vi "Template - Labview.vi"() -> ()   [LabVIEW 2017]
panel:
  out "Tempo\nTOTAL":string
  out "Tempo\nValidação":string
  out "Tempo\n Torno":string
  out "Tempo \nArmazem":string
  out "Y_Ctrg":bool
  out "Z_Ctrg":bool
  out "X_Ctrg":bool
  out "Y 1":bool
  out "Y 0":bool
  out "Z3":bool
  out "Z2":bool
  out "Z1":bool
  out "Z0":bool
  out "X 3":bool
  out "X 2":bool
  out "X 1":bool
  out "X 0":bool
  out "Medição Peça":string
  out "OK":bool
  out "Nok":bool
  out "Status":bool
  out "Robô":bool
  out "Torno":bool
  out "Visão":bool
  out "Armazem":bool
  out "Valvula 4":bool
  out "Sensor 4":bool
  out "Valvula 1":bool
  out "Sensor 1":bool
  out "Esteira 4":bool
  out "Esteira 2":bool
  out "Esteira 3":bool
  out "Esteira 1":bool
  in  "START":bool caption="OK Button"
  in  "Blank Button 74":bool
  in  "Blank Button 73":bool
  in  "Blank Button 72":bool
  in  "Blank Button 71":bool
  in  "Blank Button 70":bool
  in  "Blank Button 69":bool
  in  "Blank Button 68":bool
  in  "Blank Button 67":bool
  in  "Blank Button 66":bool
  in  "Blank Button 65":bool
  in  "Blank Button 64":bool
  in  "Blank Button 63":bool
  in  "Blank Button 62":bool
  in  "Blank Button 61":bool
  in  "Blank Button 60":bool
  in  "Blank Button 59":bool
  in  "Blank Button 58":bool
  in  "Blank Button 57":bool
  in  "Blank Button 56":bool
  in  "Blank Button 55":bool
  in  "Blank Button 54":bool
  in  "Blank Button 53":bool
  in  "Blank Button 52":bool
  in  "Blank Button 51":bool
  in  "Blank Button 50":bool
  # "Imagem"
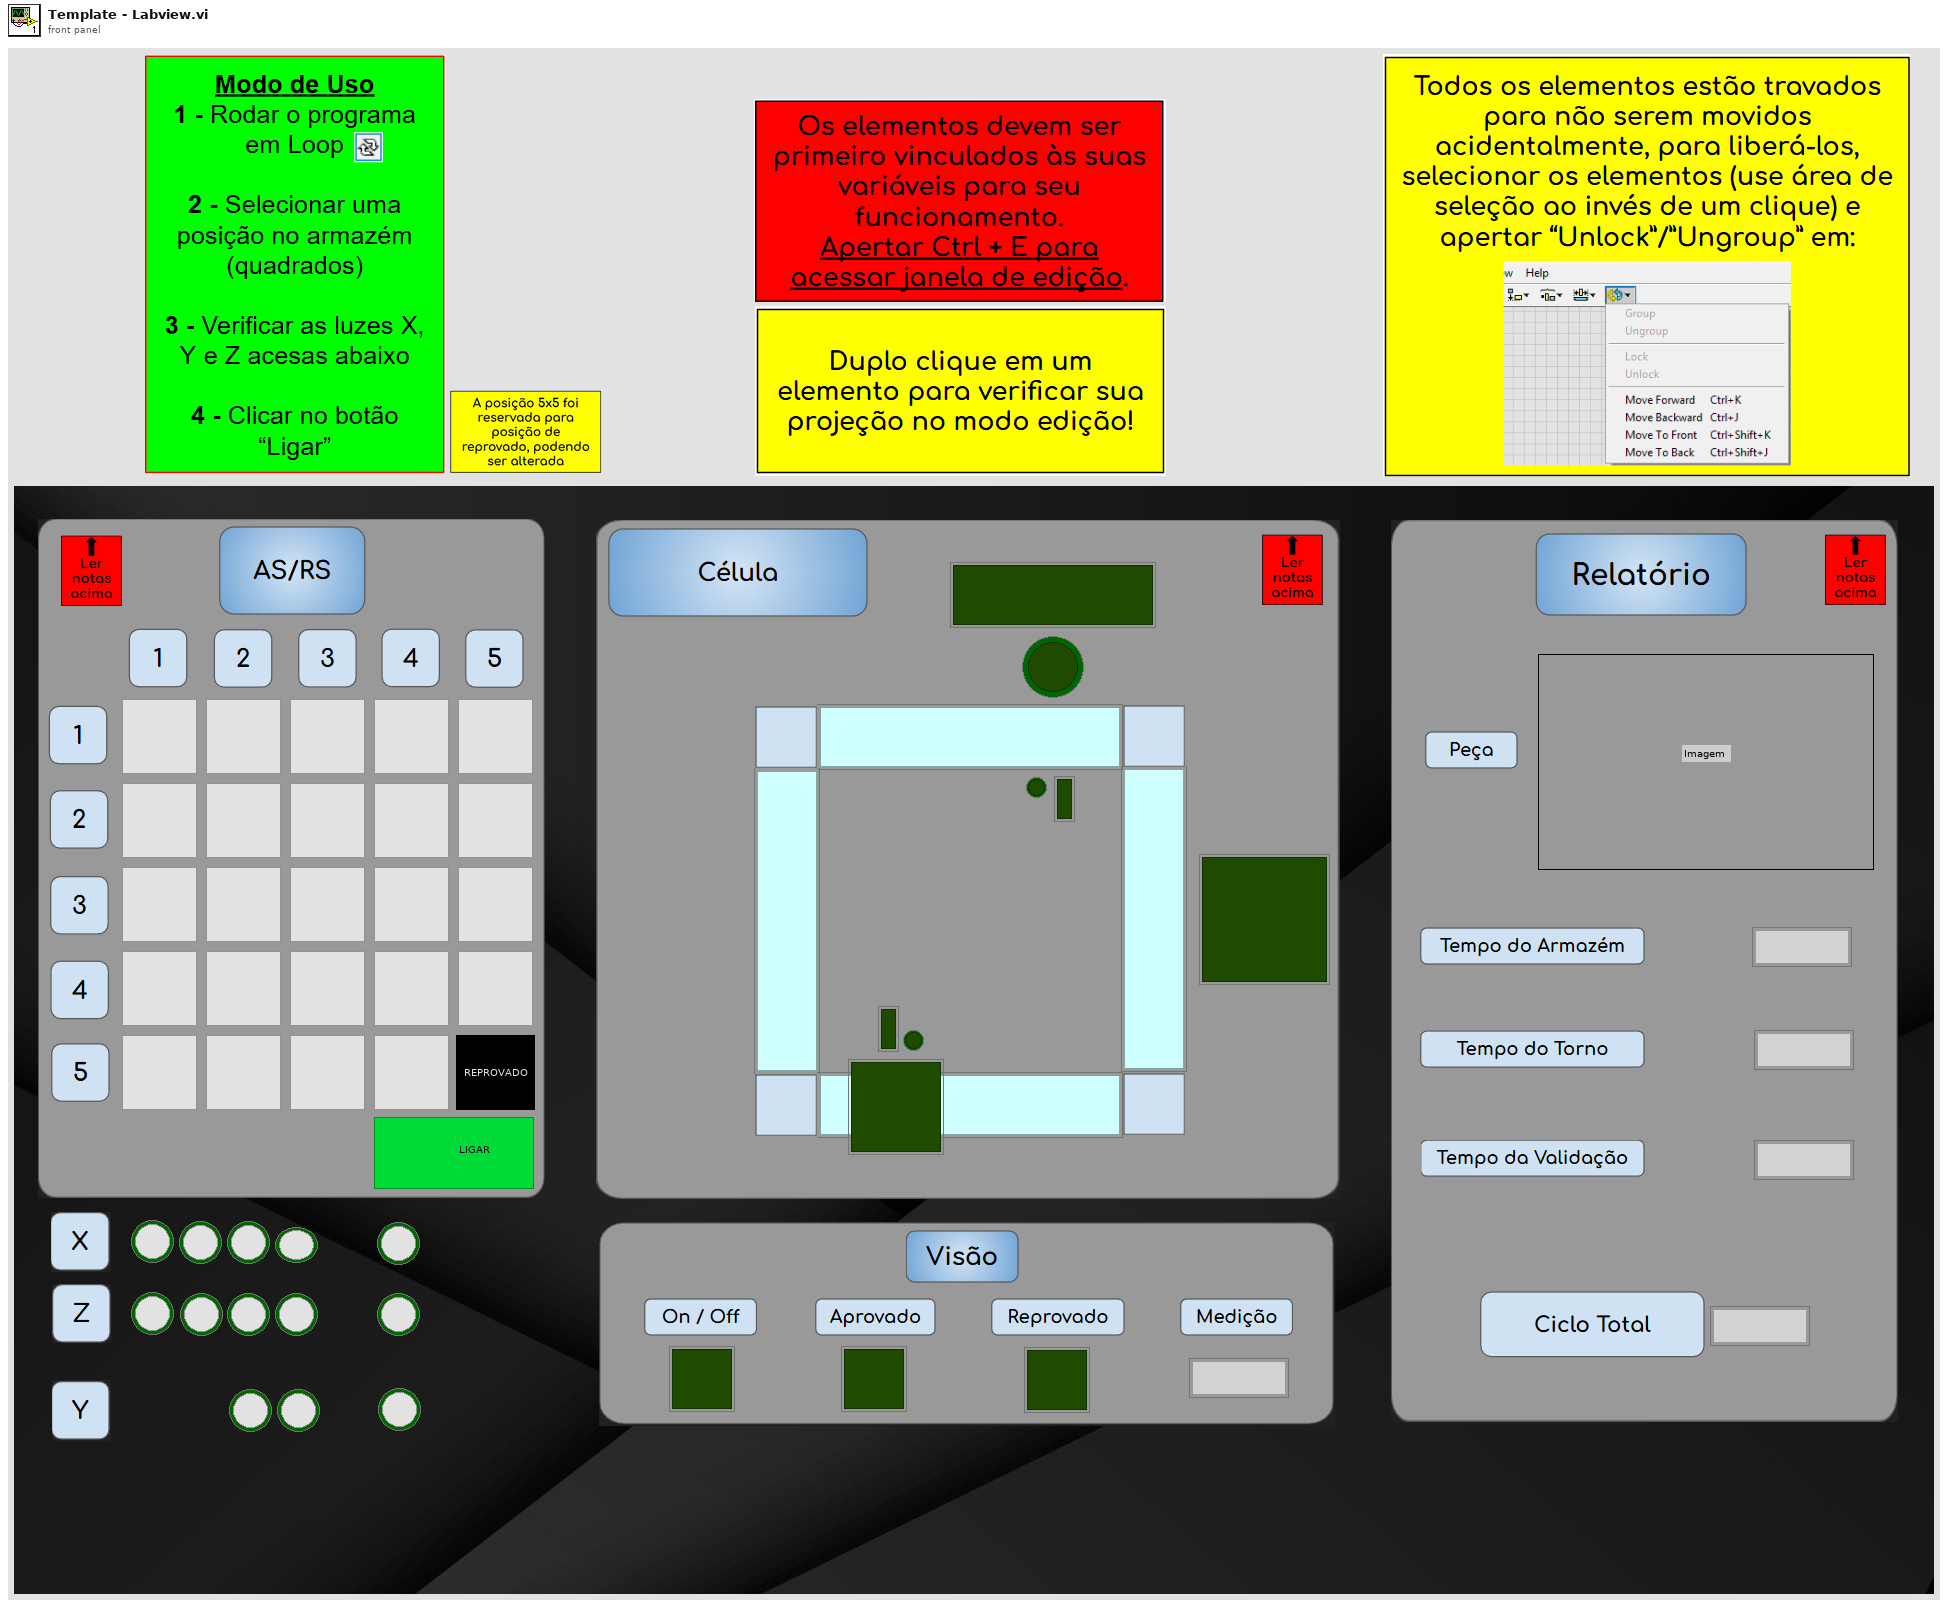
[diagram p1: front panel]
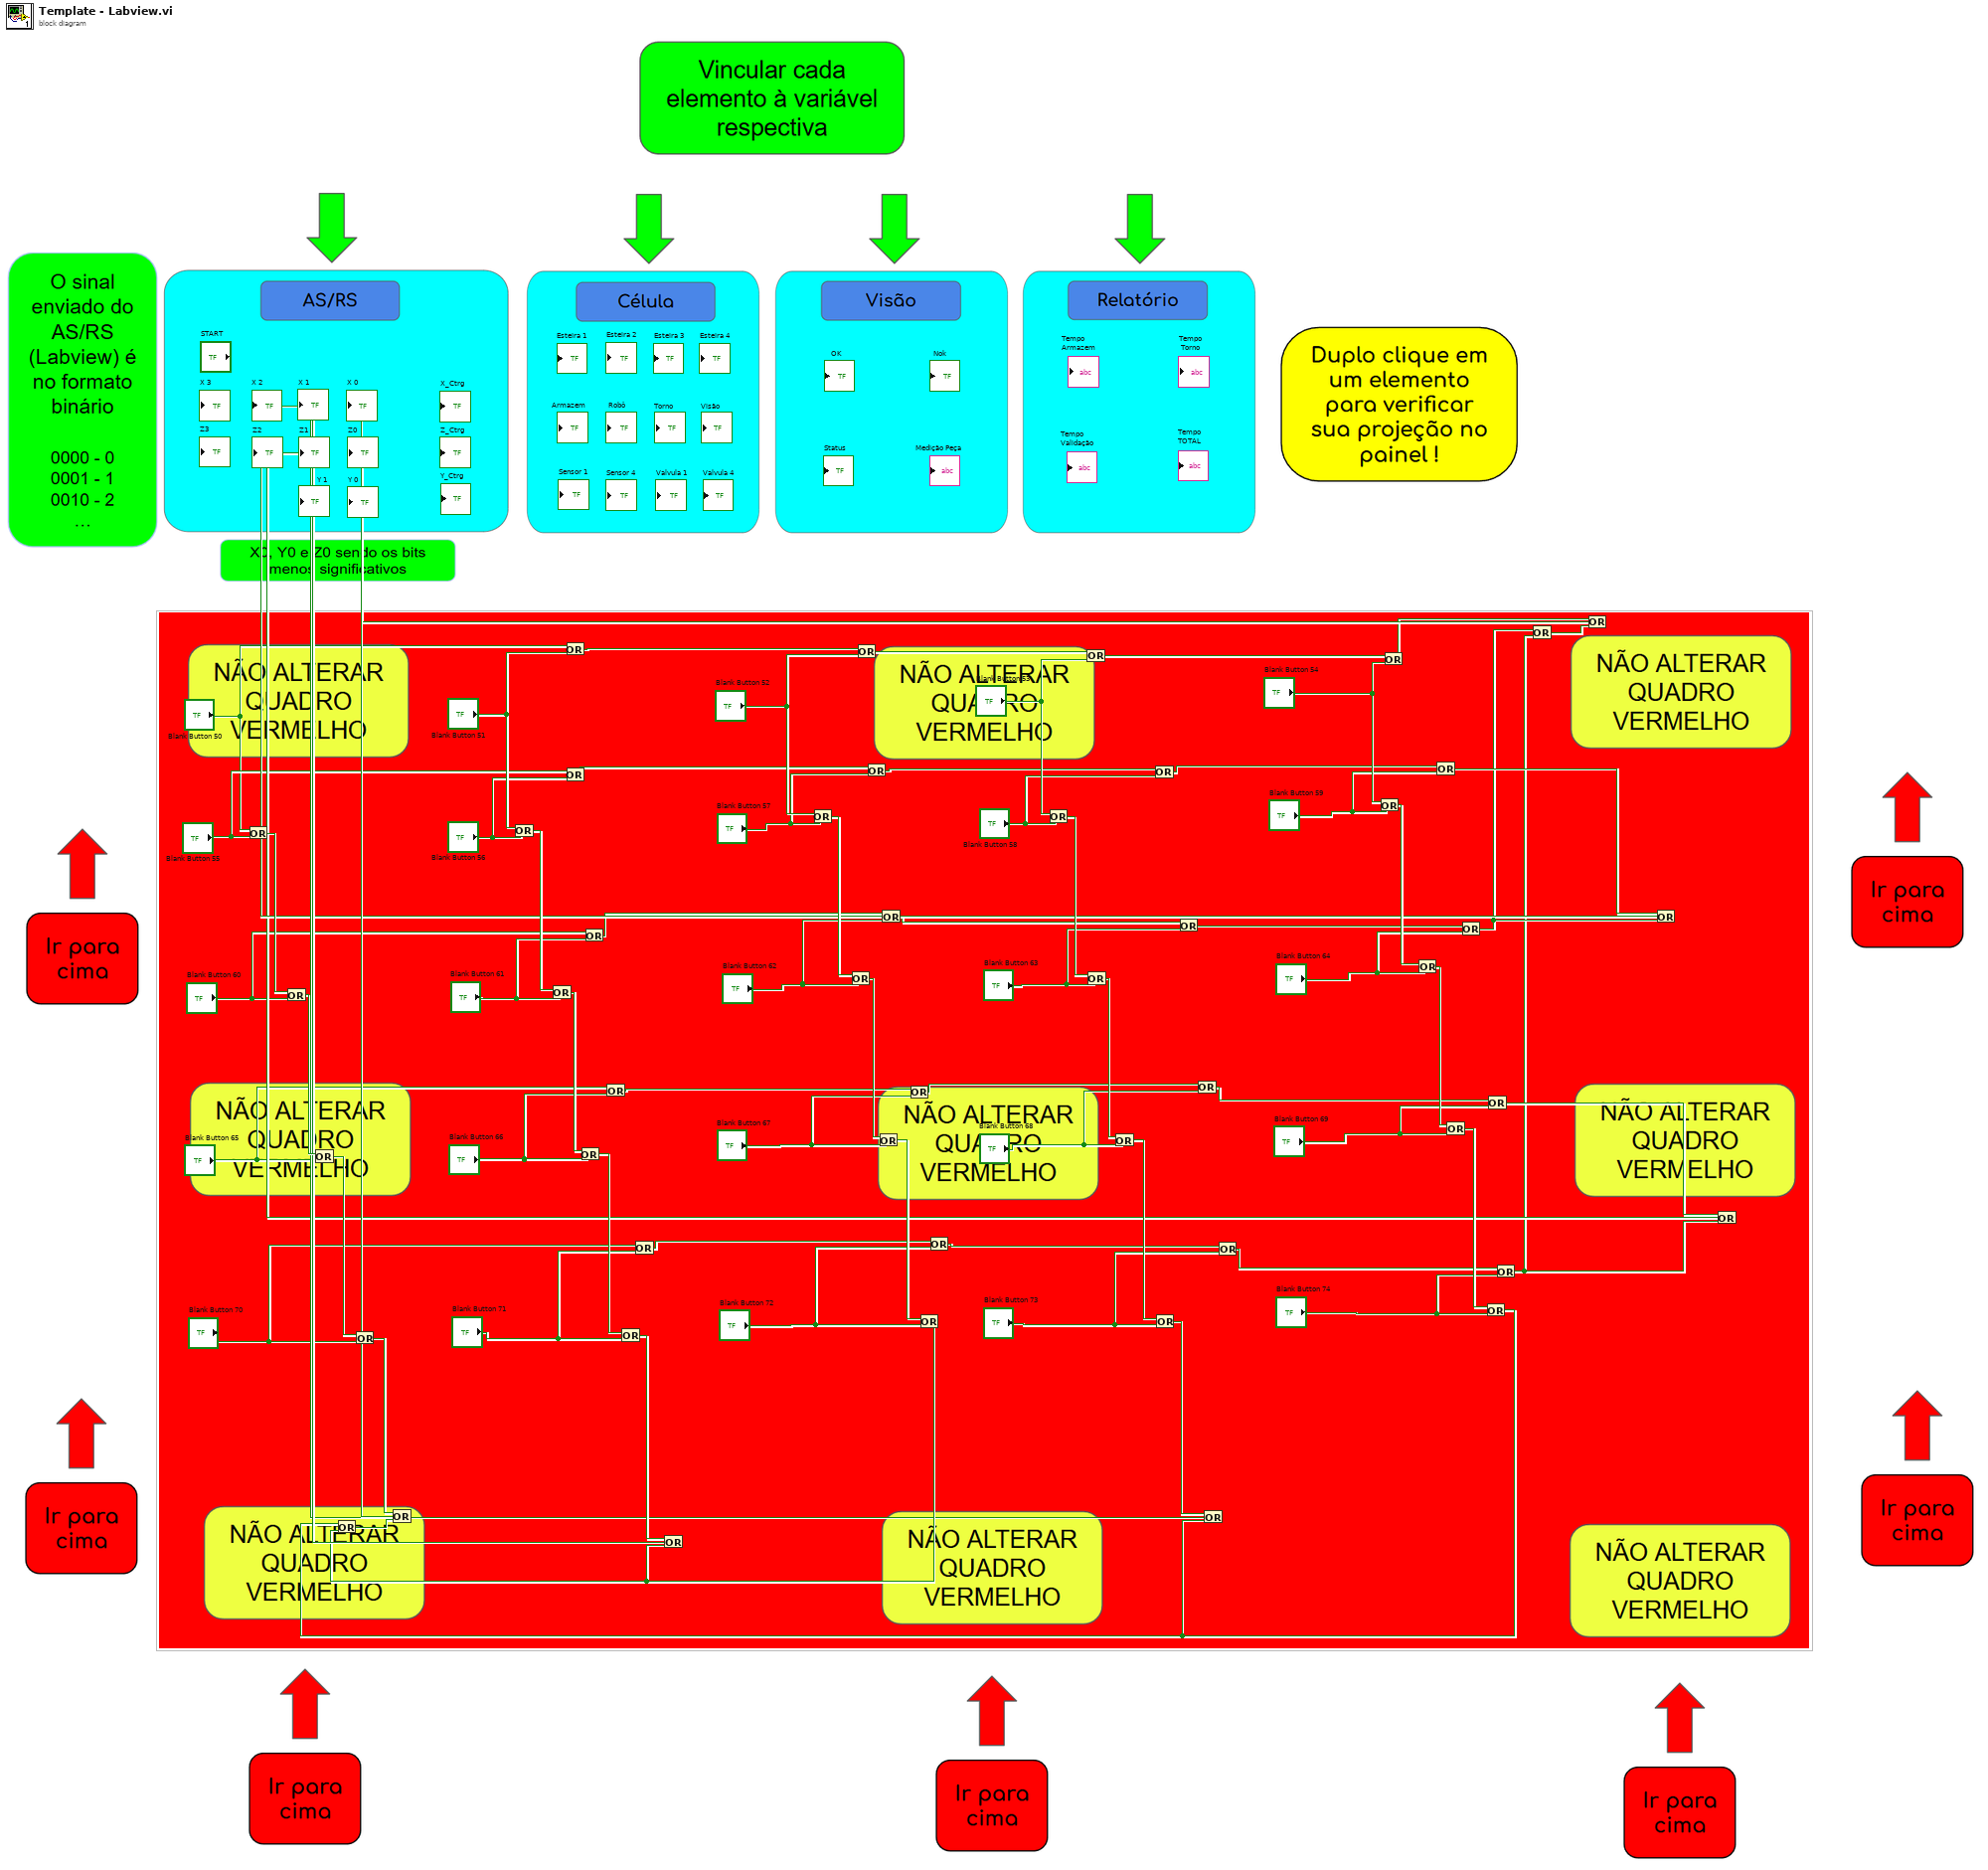
[diagram p0: block diagram]
diagram:
  n1 = Or(x="Blank Button 50", y="Blank Button 55") -> (x .or. y?=w72:bool)
  n2 = Or(x=w72, y="Blank Button 60") -> (x .or. y?=w73:bool)
  n3 = Or(x=w73, y="Blank Button 65") -> (x .or. y?=w71:bool)
  n4 = Or(x=w71, y="Blank Button 70") -> (x .or. y?=w58:bool)
  n5 = Or(x="Blank Button 51", y="Blank Button 56") -> (x .or. y?=w69:bool)
  n6 = Or(x=w69, y="Blank Button 61") -> (x .or. y?=w70:bool)
  n7 = Or(x="Blank Button 50", y="Blank Button 51") -> (x .or. y?=w44:bool)
  n8 = Or(x="Blank Button 55", y="Blank Button 56") -> (x .or. y?=w22:bool)
  n9 = Or(x=w70, y="Blank Button 66") -> (x .or. y?=w68:bool)
  n10 = Or(x="Blank Button 60", y="Blank Button 61") -> (x .or. y?=w23:bool)
  n11 = Or(x="Blank Button 65", y="Blank Button 66") -> (x .or. y?=w24:bool)
  n12 = Or(x=w68, y="Blank Button 71") -> (x .or. y?=w56:bool)
  n13 = Or(x="Blank Button 70", y="Blank Button 71") -> (x .or. y?=w25:bool)
  n14 = Or(x="Blank Button 52", y="Blank Button 57") -> (x .or. y?=w66:bool)
  n15 = Or(x=w66, y="Blank Button 62") -> (x .or. y?=w67:bool)
  n16 = Or(x=w44, y="Blank Button 52") -> (x .or. y?=w42:bool)
  n17 = Or(x=w22, y="Blank Button 57") -> (x .or. y?=w21:bool)
  n18 = Or(x=w67, y="Blank Button 67") -> (x .or. y?=w65:bool)
  n19 = Or(x=w23, y="Blank Button 62") -> (x .or. y?=w18:bool)
  n20 = Or(x=w24, y="Blank Button 67") -> (x .or. y?=w17:bool)
  n21 = Or(x=w65, y="Blank Button 72") -> (x .or. y?=w55:bool)
  n22 = Or(x=w56, y=w55) -> (x .or. y?=→"X 1":bool)
  n23 = Or(x=w25, y="Blank Button 72") -> (x .or. y?=w15:bool)
  n24 = Or(x="Blank Button 53", y="Blank Button 58") -> (x .or. y?=w63:bool)
  n25 = Or(x=w42, y="Blank Button 53") -> (x .or. y?=w40:bool)
  n26 = Or(x=w63, y="Blank Button 63") -> (x .or. y?=w64:bool)
  n27 = Or(x=w64, y="Blank Button 68") -> (x .or. y?=w62:bool)
  n28 = Or(x=w21, y="Blank Button 58") -> (x .or. y?=w6:bool)
  n29 = Or(x=w62, y="Blank Button 73") -> (x .or. y?=w51:bool)
  n30 = Or(x=w18, y="Blank Button 63") -> (x .or. y?=w8:bool)
  n31 = Or(x=w17, y="Blank Button 68") -> (x .or. y?=w10:bool)
  n32 = Or(x=w15, y="Blank Button 73") -> (x .or. y?=w12:bool)
  n33 = Or(x="Blank Button 54", y="Blank Button 59") -> (x .or. y?=w60:bool)
  n34 = Or(x=w40, y="Blank Button 54") -> (x .or. y?=w38:bool)
  n35 = Or(x=w60, y="Blank Button 64") -> (x .or. y?=w61:bool)
  n36 = Or(x=w6, y="Blank Button 59") -> (x .or. y?=w5:bool)
  n37 = Or(x=w61, y="Blank Button 69") -> (x .or. y?=w59:bool)
  n38 = Or(x=w8, y="Blank Button 64") -> (x .or. y?=w4:bool)
  n39 = Or(x=w59, y="Blank Button 74") -> (x .or. y?=w50:bool)
  n40 = Or(x=w50, y=w55) -> (x .or. y?=w54:bool)
  n41 = Or(x=w58, y=w54) -> (x .or. y?=→"X 0":bool)
  n42 = Or(x=w51, y=w50) -> (x .or. y?=→"X 2":bool)
  n43 = Or(x=w10, y="Blank Button 69") -> (x .or. y?=w3:bool)
  n44 = Or(x=w12, y="Blank Button 74") -> (x .or. y?=w2:bool)
  n45 = Or(x=w4, y=w2) -> (x .or. y?=w48:bool)
  n46 = Or(x=w38, y=w48) -> (x .or. y?=→"Z0":bool)
  n47 = Or(x=w5, y=w4) -> (x .or. y?=→"Z1":bool)
  n48 = Or(x=w3, y=w2) -> (x .or. y?=→"Z2":bool)
